vi "RD Enum Device Count.vi"(8 "error in (no error)":errorcluster caption="错误输入（无错误）", 11 "count":u32) -> (0 "error out":errorcluster caption="错误输出", 2 "function return":i32, 3 "count out":u32)   [LabVIEW 2018, in "InstrumentsPlayground.lvlib"]
doc: "CLIFFAPI int CliffEnumDeviceCount(DWORD * count);"
uses:
  InstrumentsPlayground.lvlib
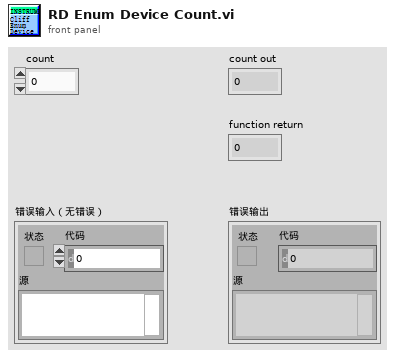
[diagram p1: front panel]
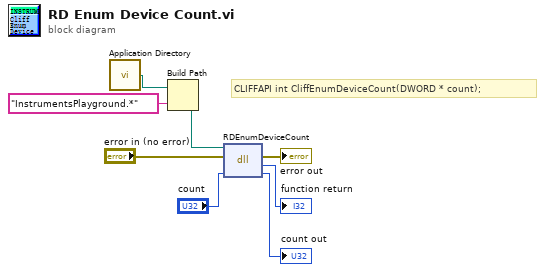
[diagram p0: block diagram]
diagram:
  # "CLIFFAPI int CliffEnumDeviceCount(DWORD * count);"
  n1 = call <vilib>:"Application Directory.vi"() -> ("Application Directory"=w2:path)
  n2 = Build Path(base path=w2, name or relative path="InstrumentsPlayground.*" ("名称或相对路径")) -> (appended path=w1:path)
  n3 = dll-call lib="E:/work/YZCourse_Xtext/Cliff/API/LabVIEW lib/InstrumentsPlayground.*" fn="RDEnumDeviceCount"(path in=w1, error in="error in (no error)", "count"="count") -> (error out=→"error out":errorcluster, "返回类型"=→"function return":i32, "count"=→"count out":u32)  [unwired: 1 in, 1 out]
